vi "3D-SaveOtherParamsConfig.vi"(7 "section":string="VISA Params", 9 "Values":string[](array[string]), 10 "Keys":string[](array[string])=["IN Stack Barcode VISA Name", "IN Stack Barcode BaudRate", "IN Stack Barcode DataBits", "IN Stack Weigh VISA Name", "IN Stack Weigh BaudRate", "IN Stack Weigh DataBits", "OUT Stack Barcode VISA Name", "OUT Stack Barcode BaudRate", "OUT Stack Barcode DataBits", "OUT Stack Weigh VISA Name", "OUT Stack Weigh BaudRate", "OUT Stack Weigh DataBits"], 11 "名称或相对路径":string="UserDefine.ini") -> ()   [LabVIEW 2017]
uses:
  Global System.vi
  <vilib>/Utility/config.llb/NI_LVConfig.lvlib
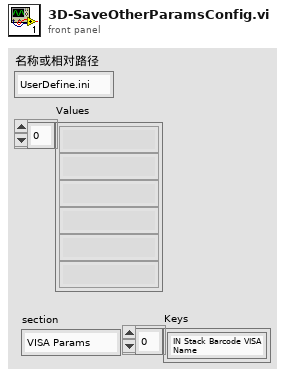
[diagram p1: front panel]
types:
  T1 = typedef "NI_LVConfig.lvlib/Config Data RefNum.ctl" = refnum<k1>
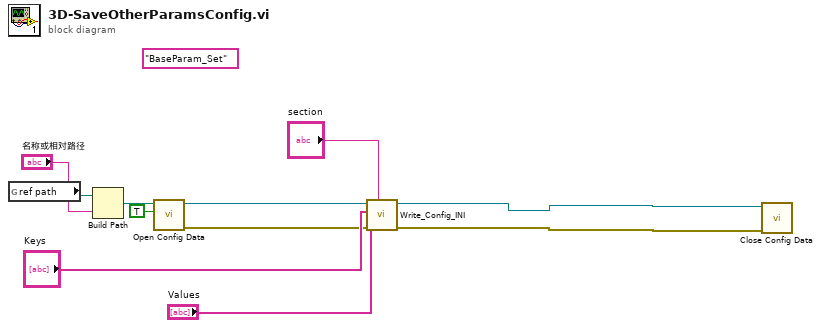
[diagram p0: block diagram]
diagram:
  (unwired) "BaseParam_Set" ("section")
  n1 = global read "Global System.vi" "ref path"() -> (w9:path)
  n2 = Build Path(base path=w9, name or relative path="名称或相对路径") -> (appended path=w8:path)
  n3 = call <vilib>:"Open Config Data.vi"("create file if necessary (T)"=TRUE, "configuration file path"=w8) -> ("error out"=w1:errorcluster, "refnum"=w2:T1)  [unwired: 7 in, 1 out]
  n4 = call "Write_Config_INI.vi"("section"="section", "error in (no error)"=w1, "Inputs"="Values", "Keys"="Keys", "refnum"=w2) -> ("error out"=w4:errorcluster, "refnum 2"=w5:T1)  [unwired: 5 in]
  n5 = call <vilib>:"Close Config Data.vi"("error in (no error)"=w4, "refnum"=w5) -> ()  [unwired: 8 in, 2 out]
